vi "FeedbackNode.vi"() -> ()   [LabVIEW 2019]
panel:
  in  "Numeric 2":i32
  out "Factorial 2":i32
  out "Factorial":i32
  in  "Numeric":i32
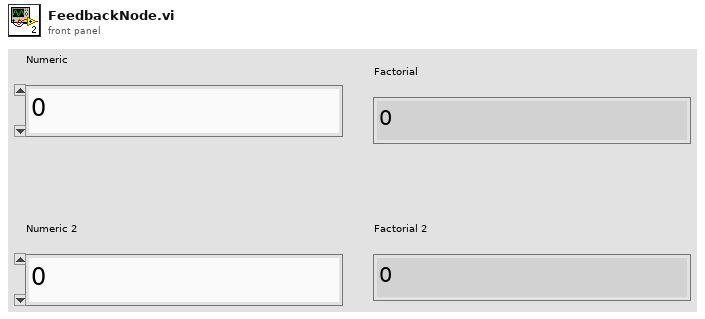
[diagram p1: front panel]
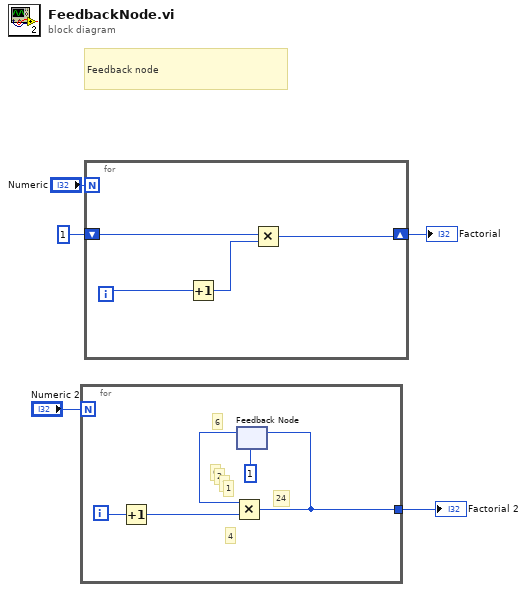
[diagram p0: block diagram]
diagram:
  # "Feedback node"
  n1 = for {
    N: "Numeric 2" -> [_]
    tunnel: [w6] -> w1
    i -> [w10]
    # "6"
    # "2"
    # "1"
    # "6"
    # "24"
    # "4"
    # "1"
    n2 = Increment(x=w10) -> (x+1=w9:i32)
    n3 = feedback #1(1) -> (w8:i32)
    n4 = Multiply(x=w8, y=w9) -> (x*y=w6:i32)
    n5 = feedback-in #1(w6) -> ()
  }
  "Factorial 2" <- w1
  n6 = for {
    N: "Numeric" -> [_]
    shift-right: [w11] -> w3
    shift-left: 1 -> [w13]
    i -> [w14]
    n7 = Increment(x=w14) -> (x+1=w12:i32)
    n8 = Multiply(x=w13, y=w12) -> (x*y=w11:i32)
  }
  "Factorial" <- w3
